vi "Substring.vi"() -> ()   [LabVIEW 2023]
panel:
  out "String 2":string
  in  "String":string
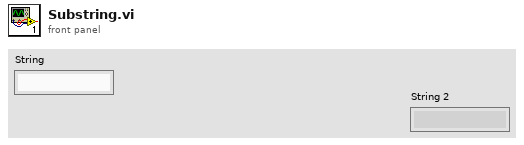
[diagram p1: front panel]
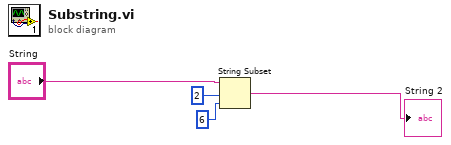
[diagram p0: block diagram]
diagram:
  n1 = String Subset(string="String", offset (0)=2, length (rest)=6) -> (substring=→"String 2":string)
